vi "Find Test Cases in lvlib.vi"(8 "error in (no error)":errorcluster, 11 "Project Path":path) -> (0 "error out":errorcluster, 2 "Test Class paths":path[](array[path]))   [LabVIEW 2020, in "Test Finder.lvclass"]
uses:
  Test Finder.lvclass
  Test Finder.lvclass/Test Finder.ctl
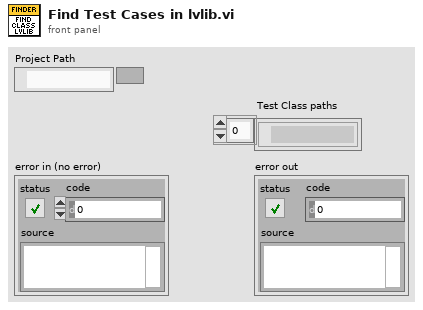
[diagram p1: front panel]
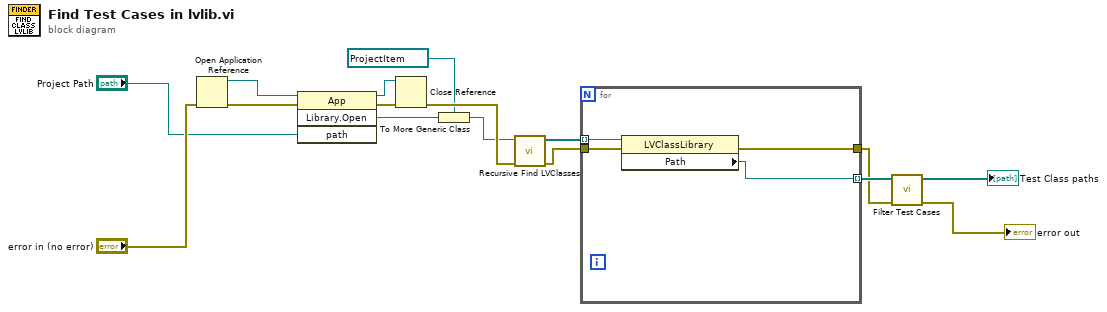
[diagram p0: block diagram]
diagram:
  n1 = Open Application Reference(8:"error in (no error)") -> (0:w12:errorcluster, 3:w11:refnum<vi>)  [unwired: 3 in]
  n2 = invoke class="App" method="Library.Open"(reference=w11, error in=w12, "path"="Project Path") -> (reference out=w14:refnum<vi>, error out=w13:errorcluster, "Open Library"=w6:refnum<vi>)  [unwired: 1 in, 1 out]
  n3 = Close Reference(reference=w14, error in (no error)=w13) -> (error out=w8:errorcluster)
  n4 = To More Generic Class(target class=refnum<vi> refnum ("reference"), reference=w6) -> (generic class reference=w5:refnum<vi>)
  n5 = call "Recursive Find LVClasses.vi"("error in (no error)"=w8, "reference"=w5) -> ("error out"=w9:errorcluster, "Class References"=w15:refnum<vi>[])  [unwired: 8 in]
  n6 = for {
    tunnel: w15 -> [w20] mode=indexing
    tunnel: w9 -> [w19]
    tunnel: [w18] -> w2
    tunnel: [w17] -> w4 mode=indexing
    n7 = property class="LVClassLibrary"(reference=w20, error in=w19) -> (error out=w18:errorcluster, "Path"=w17:path)  [unwired: 1 out]
  }
  n8 = call "Filter Test Cases.vi"("error in (no error)"=w2, "Classes to Filter"=w4) -> ("error out"=→"error out":errorcluster, "Filtered Classes"=→"Test Class paths":path[])  [unwired: 8 in]
